vi "JS_ArraytoCluster.vi"(11 "Joint States":T1(array[cluster])) -> (3 "Joint Positions 2":T2 {"left_w2" scale=-180.0..180.0; "left_w1" scale=-180.0..180.0; "left_w0" scale=-180.0..180.0; "left_e1" scale=-180.0..180.0; "left_e0" scale=-180.0..180.0; "left_s1" scale=-180.0..180.0; "left_s0" scale=-180.0..180.0; "right_s1" scale=-180.0..180.0; "right_s0" scale=-180.0..180.0; "right_w2" scale=-180.0..180.0; "right_e1" scale=-180.0..180.0; "right_e0" scale=-180.0..180.0; "right_w0" scale=-180.0..180.0; "right_w1" scale=-180.0..180.0})   [LabVIEW 2012]
uses:
  <userlib>/ROSforLV/ROS/Code/JointPositions.ctl
  <userlib>/ROSforLV/ROS/Code/Slider.ctl
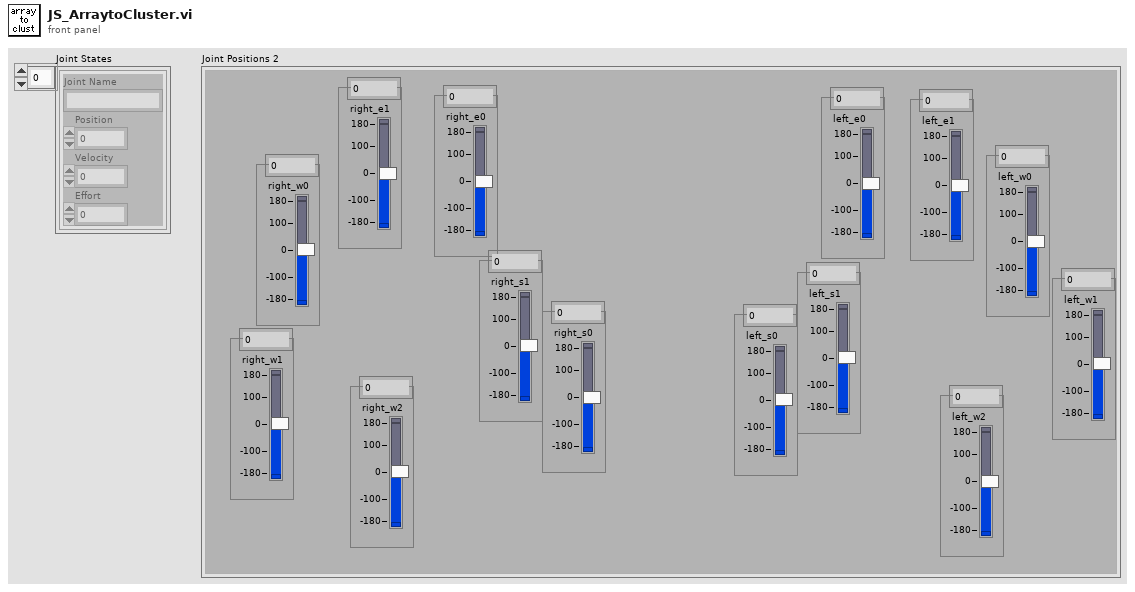
[diagram p1: front panel]
types:
  T1 = cluster{"Joint Name":string, "Position":dbl, "Velocity":dbl, "Effort":dbl}[]
  T2 = typedef "JointPositions.ctl" = cluster{"left_e0":T3, "left_e1":T3, "left_s0":T3, "left_s1":T3, "left_w0":T3, "left_w1":T3, "left_w2":T3, "right_e0":T3, "right_e1":T3, "right_s0":T3, "right_s1":T3, "right_w0":T3, "right_w1":T3, "right_w2":T3}
  T3 = typedef "Slider.ctl" = dbl
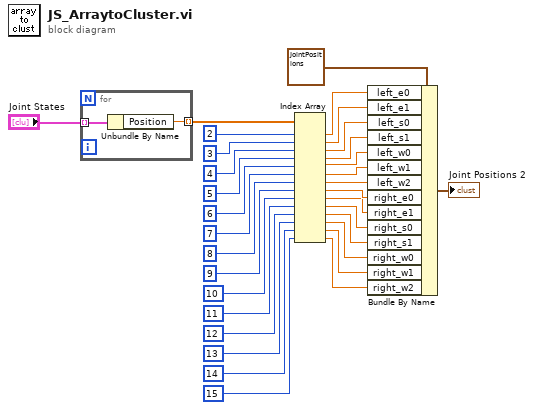
[diagram p0: block diagram]
diagram:
  n1 = for {
    tunnel: "Joint States" -> [w34] mode=indexing
    tunnel: [w33] -> w22 mode=indexing
    n2 = Unbundle By Name(w34) -> ("Position"=w33:dbl)
  }
  n3 = Index Array(array=w22, index #1=2 ("index"), index #2=3 ("index"), index #3=4 ("index"), index #4=5 ("index"), index #5=6 ("index"), index #6=7 ("index"), index #7=8 ("index"), index #8=9 ("index"), index #9=10 ("index"), index #10=11 ("index"), index #11=12 ("index"), index #12=13 ("index"), index #13=14 ("index"), index #14=15 ("index")) -> (element #1=w14:dbl, element #2=w13:dbl, element #3=w12:dbl, element #4=w11:dbl, element #5=w10:dbl, element #6=w9:dbl, element #7=w8:dbl, element #8=w7:dbl, element #9=w6:dbl, element #10=w5:dbl, element #11=w4:dbl, element #12=w3:dbl, element #13=w2:dbl, element #14=w1:dbl)
  n4 = Bundle By Name(cluster=T2 {"left_e0"=0.0, "left_e1"=0.0, "left_s0"=0.0, "left_s1"=0.0, "left_w0"=0.0, "left_w1"=0.0, "left_w2"=0.0, "right_e0"=0.0, "right_e1"=0.0, "right_s0"=0.0, "right_s1"=0.0, "right_w0"=0.0, "right_w1"=0.0, "right_w2"=0.0} ("Joint Positions 2"), "left_e0"=w14, "left_e1"=w13, "left_s0"=w12, "left_s1"=w11, "left_w0"=w10, "left_w1"=w9, "left_w2"=w8, "right_e0"=w7, "right_e1"=w6, "right_s0"=w5, "right_s1"=w4, "right_w0"=w3, "right_w1"=w2, "right_w2"=w1) -> (→"Joint Positions 2":T2)
